vi "1820_Calculate_Sweep_Time.vi"(8 "Power Supply Field (T)":dbl, 9 "Target Field Rate (T/min)":dbl, 10 "Magnet Field (T)":dbl, 11 "Target Field (T)":dbl) -> (1 "Remaining Time (min)":dbl, 3 "ETA":timestamp)   [LabVIEW 2016]
uses:
  API/Mercury-1820-API.lvlib
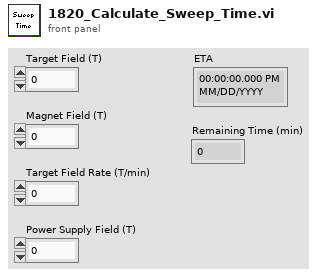
[diagram p1: front panel]
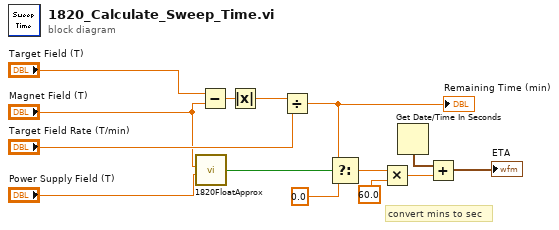
[diagram p0: block diagram]
diagram:
  # "convert mins to sec"
  n1 = call "1820FloatApprox.vi"("y"="Power Supply Field (T)", "x"="Magnet Field (T)") -> ("x ~ y?"=w7:bool)  [unwired: 2 in]
  n2 = Subtract(x="Target Field (T)", y="Magnet Field (T)") -> (x-y=w9:dbl)
  n3 = Absolute Value(x=w9) -> (abs(x)=w1:dbl)
  n4 = Divide(x=w1, y="Target Field Rate (T/min)") -> (x/y=w12:dbl)
  "Remaining Time (min)" <- w12
  n5 = Select(t=w12, s=w7, f=0.0) -> (s? t:f=w4:dbl)
  n6 = Multiply(x=w4, y=60.0 ("f")) -> (x*y=w3:dbl)
  n7 = Get Date/Time In Seconds() -> (seconds since 1Jan1904=w6:timestamp)
  n8 = Add(x=w6, y=w3) -> (x+y=→"ETA":timestamp)
